vi "subMFD_CoefQuant & Analysis.vi"() -> ()   [LabVIEW 2023]
uses:
  <vilib>/addons/Digital Filter Design/_Objects.llb/DFD Multirate Filter Obj.ctl
  <vilib>/addons/Digital Filter Design/_Objects.llb/DFD Multirate Mode.ctl
  <vilib>/addons/Digital Filter Design/_Objects.llb/DFD Coef Norm Type.ctl
  <vilib>/addons/Digital Filter Design/_Objects.llb/DFD Round-off Mode.ctl
  <vilib>/addons/Digital Filter Design/_Objects.llb/DFD FXP MRate Multiply Mode.ctl
  <vilib>/addons/Digital Filter Design/_Objects.llb/DFD Phase Setting.ctl
  <vilib>/addons/Digital Filter Design/NI_DigFilterLicensed.lvlib
panel:
  out "Postprocessing Gain":dbl=nan min=1.0 max=32.0 step=1.0 format="%#_4e"
  in  "Gain Word Length":i16=16 min=2 max=32 step=1
  in  "Gain Processing":u16(ring)=1 items=["On Target", "On Host"]
  in  "Scale Type":u16(ring)=1 items=["No Norm", "Time Domain 1-Norm", "Time Domain 2-Norm", "Time Domain Inf-Norm"]
  in  "Scale by Power of 2?":bool
  in  "Coefficients Word Length":i16=16 min=1 max=32 step=1
  out "Successful Design?":bool
  out "multirate filter out":T1={"mMRate_Structure"=enum."FIR", "mMRate_Mode"=0, "mMRate_Factor"=-1, "mMRate_FIRParams"={"mMRate_FIR_H"=[], "mMRate_FIR_IsNyquist?"=FALSE, "mMRate_FIR_IsSymmetric?"=FALSE}, "mMRate_CICParams"={"mMRate_CIC_#Stage"=0, "mMRate_CIC_Lag"=1, "mMRate_CIC_Type"=enum."Lowpass"}, "mMRate_Order"=0, "mMRate_Version"="2.0", "mMRate_Comments"="", "mMRate_RationalFactor"={"mMRate_L"=-1, "mMRate_M"=-1}, "mMRate_Fs"=1.0, "mMRate_Quantized?"=FALSE, "mMRate_QFilterGain"=1.0, "mMRate_CoefWl"=16, "mMRate_Scaling"={"mMRate_ScaleByPowerOf2?"=FALSE, "mMRate_ScaleType"=enum."No Norm"}, "mMRate_InputWl"=16, "mMRate_OutputWl"=16, "mMRate_OutputMode"=enum."Truncation", "mMRate_MultMode"=enum."Truncated", "mMRate_BitPruning"=FALSE, "mMRate_GainWl"=16, "mMRate_OutputFwl"=0, "mMRate_SumIwl"=0, "mMRate_InputIwl "=16, "mMRate_SumWl"=32, "mMRate_CoefIwl"=0} {"mMRate_SumWl" min=1 max=32 step=1; "mMRate_InputIwl" min=1 max=32 step=1; "mMRate_GainWl" min=1 max=32 step=1; "mMRate_OutputWl" min=1 max=32 step=1; "mMRate_InputWl" min=1 max=32 step=1; "mMRate_CoefWl" min=1 max=32 step=1; "mMRate_Mode" items=["Default"=-1, "No Rate Change"=0, "Interpolation"=1, "Decimation"=2, "Interpolated"=3, "Rational"=4]}
  in  "multirate filter in":T1={"mMRate_Structure"=enum."FIR", "mMRate_Mode"=0, "mMRate_Factor"=-1, "mMRate_FIRParams"={"mMRate_FIR_H"=[], "mMRate_FIR_IsNyquist?"=FALSE, "mMRate_FIR_IsSymmetric?"=FALSE}, "mMRate_CICParams"={"mMRate_CIC_#Stage"=0, "mMRate_CIC_Lag"=1, "mMRate_CIC_Type"=enum."Lowpass"}, "mMRate_Order"=0, "mMRate_Version"="2.0", "mMRate_Comments"="", "mMRate_RationalFactor"={"mMRate_L"=-1, "mMRate_M"=-1}, "mMRate_Fs"=1.0, "mMRate_Quantized?"=FALSE, "mMRate_QFilterGain"=1.0, "mMRate_CoefWl"=16, "mMRate_Scaling"={"mMRate_ScaleByPowerOf2?"=FALSE, "mMRate_ScaleType"=enum."No Norm"}, "mMRate_InputWl"=16, "mMRate_OutputWl"=16, "mMRate_OutputMode"=enum."Truncation", "mMRate_MultMode"=enum."Truncated", "mMRate_BitPruning"=FALSE, "mMRate_GainWl"=16, "mMRate_OutputFwl"=0, "mMRate_SumIwl"=0, "mMRate_InputIwl "=16, "mMRate_SumWl"=32, "mMRate_CoefIwl"=0} {"mMRate_SumWl" min=1 max=32 step=1; "mMRate_InputIwl" min=1 max=32 step=1; "mMRate_GainWl" min=1 max=32 step=1; "mMRate_OutputWl" min=1 max=32 step=1; "mMRate_InputWl" min=1 max=32 step=1; "mMRate_CoefWl" min=1 max=32 step=1; "mMRate_Mode" items=["Default"=-1, "No Rate Change"=0, "Interpolation"=1, "Decimation"=2, "Interpolated"=3, "Rational"=4]}
  in  "Graph Selector":u16(ring) items=["Magnitude", "Phase", "Coefficients"]
  in  "Unwrap?":bool=TRUE
  out "Graph Tab":enum32{"Magnitude", "Phase", "Coefficients"}(tab)
  out "Magnitude Response":cluster{"f0":dbl, "df":dbl, "values":dbl[]}[](graph)
  out "Phase Response":cluster{"f0":dbl, "df":dbl, "values":dbl[]}[](graph)
  out "Coefficients":dbl[][](graph)
  in  "Magnitude in dB?":bool=TRUE
  out "OK":bool
  in  "stop":bool
  # "Design Result"
  # "Coefficients Quantization Settings"
  # "Gain Settings"
  # "Postprocessing\nGain"
  # "Gain Processing"
  # "Gain\nWord Length"
  # "Demo Program"
  # "Coefficients\nWord Length"
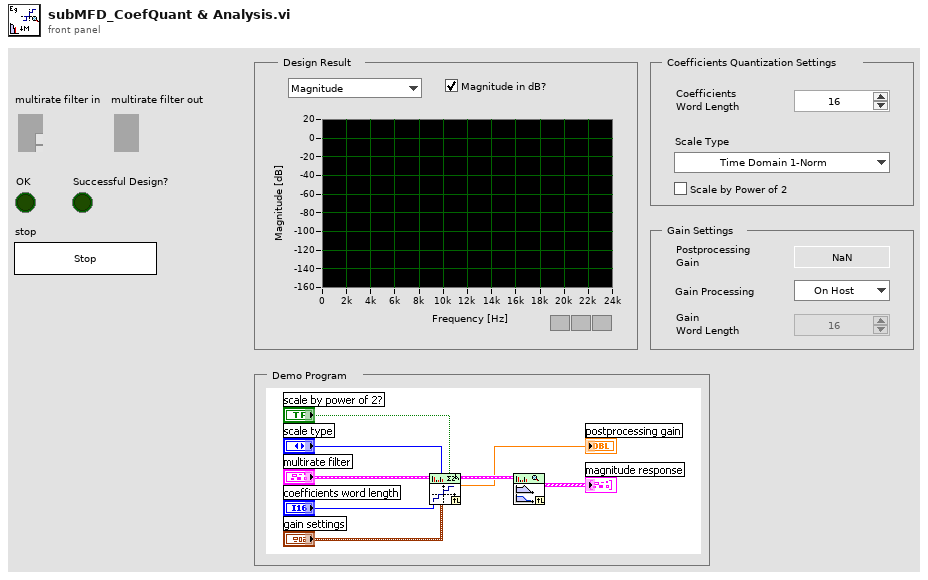
[diagram p1: front panel]
types:
  T1 = typedef "NI_DigFilterLicensed.lvlib/DFD Multirate Filter Obj.ctl" = cluster{"mMRate_Structure":enum16{"CIC", "FIR", "IIR", "Lattice"}, "mMRate_Mode":T2, "mMRate_Factor":i32, "mMRate_FIRParams":cluster{"mMRate_FIR_H":dbl[], "mMRate_FIR_IsNyquist?":bool, "mMRate_FIR_IsSymmetric?":bool}, "mMRate_CICParams":cluster{"mMRate_CIC_#Stage":i32, "mMRate_CIC_Lag":i32, "mMRate_CIC_Type":enum16{"Lowpass", "Highpass"}}, "mMRate_Order":i32, "mMRate_Version":string, "mMRate_Comments":string, "mMRate_RationalFactor":cluster{"mMRate_L":i32, "mMRate_M":i32}, "mMRate_Fs":dbl, "mMRate_Quantized?":bool, "mMRate_QFilterGain":dbl, "mMRate_CoefWl":i16, "mMRate_Scaling":cluster{"mMRate_ScaleByPowerOf2?":bool, "mMRate_ScaleType":T3}, "mMRate_InputWl":i16, "mMRate_OutputWl":i16, "mMRate_OutputMode":T4, "mMRate_MultMode":T5, "mMRate_BitPruning":bool, "mMRate_GainWl":i16, "mMRate_OutputFwl":i16, "mMRate_SumIwl":i16, "mMRate_InputIwl ":i16, "mMRate_SumWl":i16, "mMRate_CoefIwl":i16}
  T2 = typedef "NI_DigFilterLicensed.lvlib/DFD Multirate Mode.ctl" = i16
  T3 = typedef "NI_DigFilterLicensed.lvlib/DFD Coef Norm Type.ctl" = enum16{"No Norm", "Time Domain 1-Norm", "Time Domain 2-Norm", "Time Domain Inf-Norm"}
  T4 = typedef "NI_DigFilterLicensed.lvlib/DFD Round-off Mode.ctl" = enum16{"Nearest", "Truncation"}
  T5 = typedef "NI_DigFilterLicensed.lvlib/DFD FXP MRate Multiply Mode.ctl" = enum16{"Truncated", "Full"}
  T6 = typedef "NI_DigFilterLicensed.lvlib/DFD Phase Setting.ctl" = cluster{"unwrap? (F)":bool, "degree? (F)":bool}
  T7 = cluster{"Gain Processing":u16, "Gain Word Length":i16}
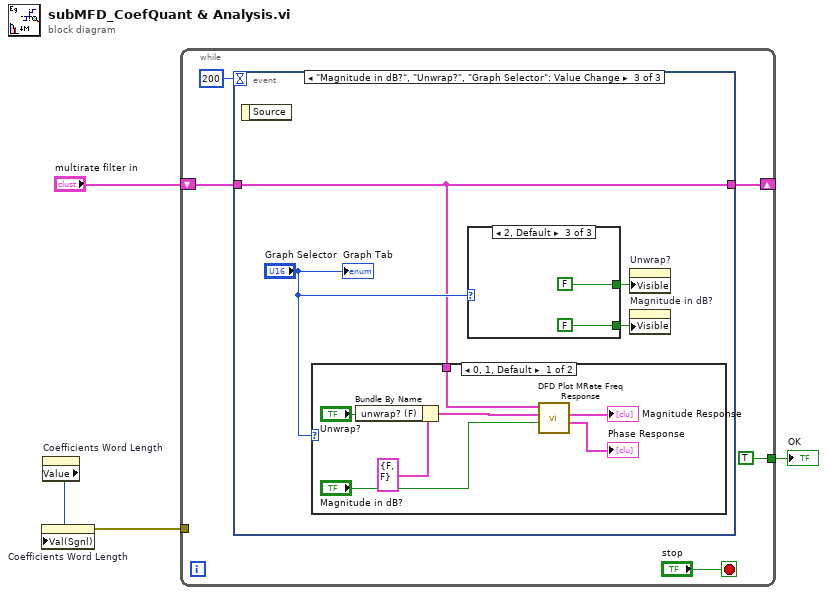
[diagram p0: block diagram]
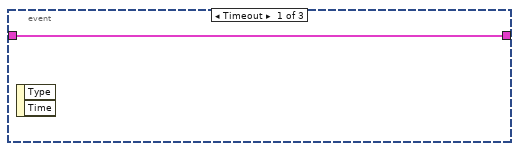
[diagram p2: hidden frame]
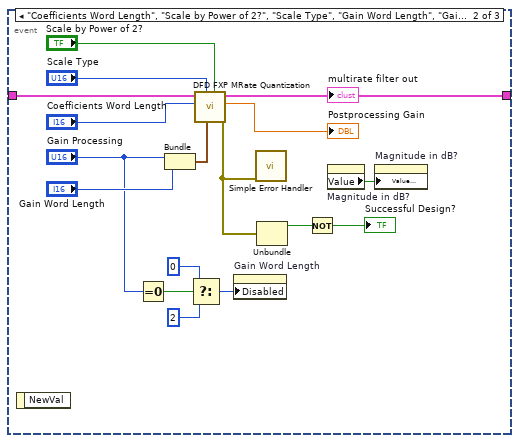
[diagram p3: hidden frame]
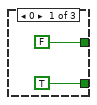
[diagram p4: hidden frame]
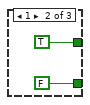
[diagram p5: hidden frame]
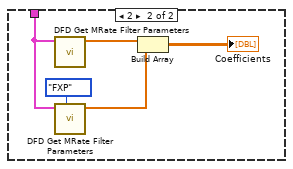
[diagram p6: hidden frame]
diagram:
  n1 = property on="Coefficients Word Length" class="DigNum (strict)"() -> ("Value"=w2:i16)  [unwired: 2 in, 2 out]
  n2 = property on="Coefficients Word Length" class="DigNum (strict)"("Val(Sgnl)"=w2) -> (error out=w3:errorcluster)  [unwired: 2 in, 1 out]
  n3 = while {
    tunnel: [TRUE] -> w4
    shift-right: [w5] -> _
    shift-left: "multirate filter in" -> [w6]
    tunnel: w3 -> [_]
    stop <- "stop" stop-if-true
    n4 = event shown="[2] \"Magnitude in dB?\", \"Unwrap?\", \"Graph Selector\": Value Change" {
      selector: _ -> [_ _ _]
      dyn-events: _ -> [_ _ _]
      timeout: 200 -> [_ _ _]
      tunnel: w6 -> [w10 w26 w28]
      tunnel: [w10 w22 w28] -> w5
      event Timeout {
        n5 = event-data() -> ()  [unwired: 3 out]
      }
      event "Coefficients Word Length", "Scale by Power of 2?", "Scale Type", "Gain Word Length", "Gain Processing": Value Change {
        n6 = event-data() -> ()  [unwired: 2 out]
        n7 = Equal To 0?(x="Gain Processing") -> (x = 0?=w17:bool)
        n8 = Bundle("Gain Processing"="Gain Processing", "Gain Word Length"="Gain Word Length") -> (w20:T7)  [unwired: 1 out]
        n9 = Select(t=u8 0 ("Disabled"), s=w17, f=u8 2) -> (s? t:f=w16:u8)
        n10 = call <vilib>:"DFD FXP MRate Quantization.vi"("scale by power of 2? (F)"="Scale by Power of 2?", "gain settings"=w20, "scale type"="Scale Type", "coefficients word length"="Coefficients Word Length", "multirate filter in"=w26) -> ("error out"=w13:errorcluster, "postprocessing gain"=→"Postprocessing Gain":dbl, "multirate filter out"=w22:T1)  [unwired: 1 in, 3 out]
        "multirate filter out" <- w22
        n11 = property on="Gain Word Length" class="DigNum (strict)"("Disabled"=w16) -> ()  [unwired: 2 in, 2 out]
        n12 = call <vilib>:"Simple Error Handler.vi"("error in (no error)"=w13) -> ()  [unwired: 1 in, 8 out]
        n13 = Unbundle(w13) -> ("status"=w12:bool)  [unwired: 2 out]
        n14 = Not(x=w12) -> (.not. x?=→"Successful Design?":bool)
        n15 = property on="Magnitude in dB?" class="Bool (strict)"() -> ("Value"=w27:bool)  [unwired: 2 in, 2 out]
        n16 = property on="Magnitude in dB?" class="Bool (strict)"("Value (Signaling)"=w27) -> ()  [unwired: 2 in, 2 out]
      }
      event "Magnitude in dB?", "Unwrap?", "Graph Selector": Value Change {
        n17 = event-data() -> ()  [unwired: 2 out]
        n18 = case shown="0, 1, Default" "Graph Selector" {
          tunnel: w28 -> [w38 w45]
          frame 0, 1, Default {
            n19 = Bundle By Name(cluster=T6 {"unwrap? (F)"=FALSE, "degree? (F)"=FALSE} ("phase view"), "unwrap? (F)"="Unwrap?") -> (w40:T6)
            n20 = call <vilib>:"DFD Plot MRate Freq Response.vi"("dB on? (T)"="Magnitude in dB?", "phase view"=w40, "multirate filter in"=w38) -> ("phase response"=→"Phase Response":cluster{"f0":dbl, "df":dbl, "values":dbl[]}[], "magnitude response"=→"Magnitude Response":cluster{"f0":dbl, "df":dbl, "values":dbl[]}[])  [unwired: 4 in, 3 out]
          }
          frame 2 {
            n21 = call <vilib>:"DFD Get MRate Filter Parameters.vi"("multirate filter in"=w45) -> ("h(n)"=w47:dbl[])  [unwired: 2 in, 8 out]
            n22 = call <vilib>:"DFD Get MRate Filter Parameters.vi"("type (FLP)"=enum16{"FLP", "FXP"}."FXP", "multirate filter in"=w45) -> ("h(n)"=w46:dbl[])  [unwired: 1 in, 8 out]
            n23 = Build Array(w47, w46) -> (→"Coefficients":dbl[][])
          }
        }
        n24 = case shown="2, Default" "Graph Selector" {
          tunnel: [FALSE TRUE FALSE] -> w31
          tunnel: [TRUE FALSE FALSE] -> w30
          frame 0 {
          }
          frame 1 {
          }
          frame 2, Default {
          }
        }
        n25 = property on="Unwrap?" class="Bool (strict)"("Visible"=w31) -> ()  [unwired: 2 in, 2 out]
        n26 = property on="Magnitude in dB?" class="Bool (strict)"("Visible"=w30) -> ()  [unwired: 2 in, 2 out]
        "Graph Tab" <- "Graph Selector"
      }
    }
  }
  "OK" <- w4
